vi "draw_stimulus_given_tracks.vi"(0 "Stimulus Image In":T2, 2 "Stimulus Snippet Array":T1[](array[typedef]), 3 "error in (no error)":errorcluster, 4 "CalibrationImage":T2) -> (7 "Stimulus Image Out":T2, 10 "error out":errorcluster)   [LabVIEW 2019]
uses:
  <vilib>/vision/Image Controls.llb/IMAQ Image.ctl
  StimulusSnippetCluster.ctl
  ParametersGlobal.vi
  StimulusObject.lvclass
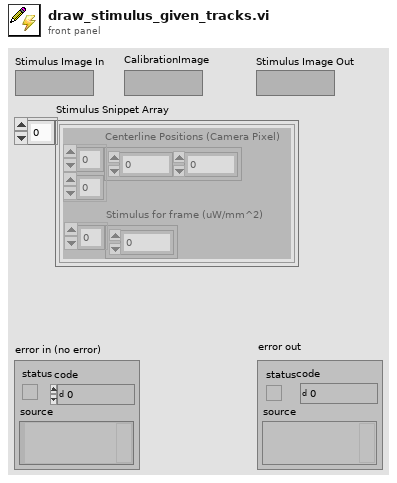
[diagram p1: front panel]
types:
  T1 = typedef "StimulusSnippetCluster.ctl" = cluster{"Centerline Positions (Camera Pixel)":sgl[][], "Stimulus for frame (uW/mm^2)":sgl[]}
  T2 = typedef "IMAQ Image.ctl" = refnum<image>
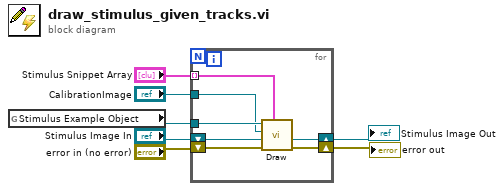
[diagram p0: block diagram]
diagram:
  n1 = global read "ParametersGlobal.vi" "Stimulus Example Object"() -> (w2:refnum<class "StimulusObject.lvclass">)
  n2 = for {
    shift-right: [w13] -> w6
    shift-left: "Stimulus Image In" -> [w14]
    shift-right: [w11] -> w4
    shift-left: "error in (no error)" -> [w12]
    tunnel: "Stimulus Snippet Array" -> [w10] mode=indexing
    tunnel: w2 -> [w9]
    tunnel: "CalibrationImage" -> [w8]
    n3 = call-dynamic "Draw.vi"("Stimulus Snippet"=w10, "error in (no error)"=w12, "StimulusImageIn"=w14, "CalibrationImage"=w8, "StimulusObject in"=w9) -> ("error out"=w11:errorcluster, "StimulusImageOut"=w13:T2)  [unwired: 4 in, 1 out]
  }
  "error out" <- w4
  "Stimulus Image Out" <- w6
